vi "Wait for Client.vi"(8 "Error In":errorcluster, 9 "userInfo":T1, 10 "workspace":T2={"x"=200.0, "y"=200.0, "z"=0.0}, 11 "Local TCP Port":u16=32123) -> (0 "Error Out":errorcluster, 3 "Connection":T3={"UDP Connection ID"=refnum, "TCP Connection ID"=refnum, "Remote UDP Port"=61557, "Remote IP"=0})   [LabVIEW 2017, in "Game.lvlib" / "GameComms.lvlib"]
uses:
  GameComms.lvlib
  TypeDefs/Connection.ctl
  TypeDefs/WorkspaceConfig.ctl
  TypeDefs/UserInfo.ctl
  TypeDefs/TCP UDP Ref FGV Commands.ctl
  TypeDefs/ClientConfigData.ctl
  TypeDefs/ClientNetworkParameters.ctl
  TypeDefs/ServerConfigData.ctl
  TypeDefs/ServerNetworkParameters.ctl
panel:
  out "net address":u32
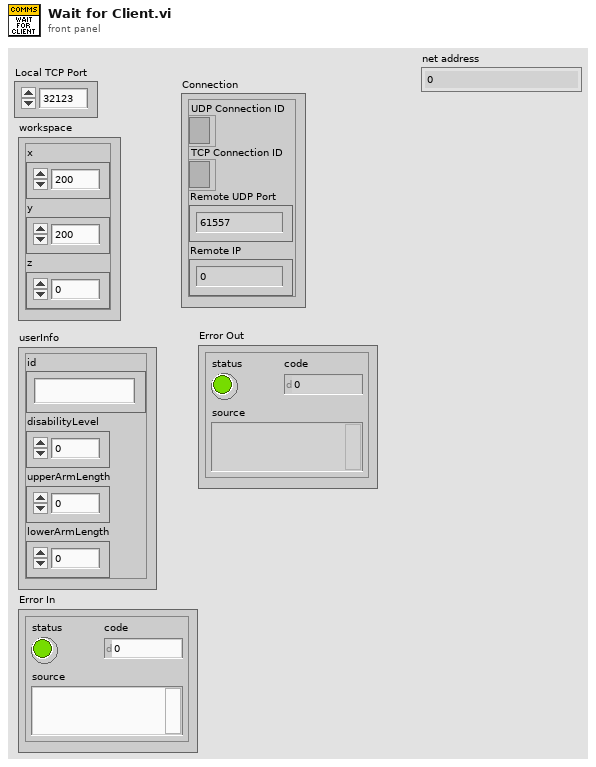
[diagram p1: front panel]
types:
  T1 = typedef "Game.lvlib/GameComms.lvlib/UserInfo.ctl" = cluster{"id":string, "disabilityLevel ":dbl, "upperArmLength":dbl, "lowerArmLength":dbl}
  T2 = typedef "Game.lvlib/GameComms.lvlib/WorkspaceConfig.ctl" = cluster{"x":dbl, "y":dbl, "z":dbl}
  T3 = typedef "Game.lvlib/GameComms.lvlib/Connection.ctl" = cluster{"UDP Connection ID":refnum<k16>, "TCP Connection ID":refnum<k5>, "Remote UDP Port":u16, "Remote IP":u32}
  T4 = enum16{"Standard", "Buffered", "CRLF", "Immediate"}
  T5 = typedef "Game.lvlib/GameComms.lvlib/ServerConfigData.ctl" = cluster{"network":T6, "workspace":T2, "userInfo":T1}
  T6 = typedef "Game.lvlib/GameComms.lvlib/ServerNetworkParameters.ctl" = cluster{"serverUdpPort":u16}
  T7 = typedef "Game.lvlib/GameComms.lvlib/ClientConfigData.ctl" = cluster{"network":T8}
  T8 = typedef "Game.lvlib/GameComms.lvlib/ClientNetworkParameters.ctl" = cluster{"clientUdpPort":u16}
  T9 = typedef "Game.lvlib/GameComms.lvlib/TCP UDP Ref FGV Commands.ctl" = enum16{"Set", "Get"}
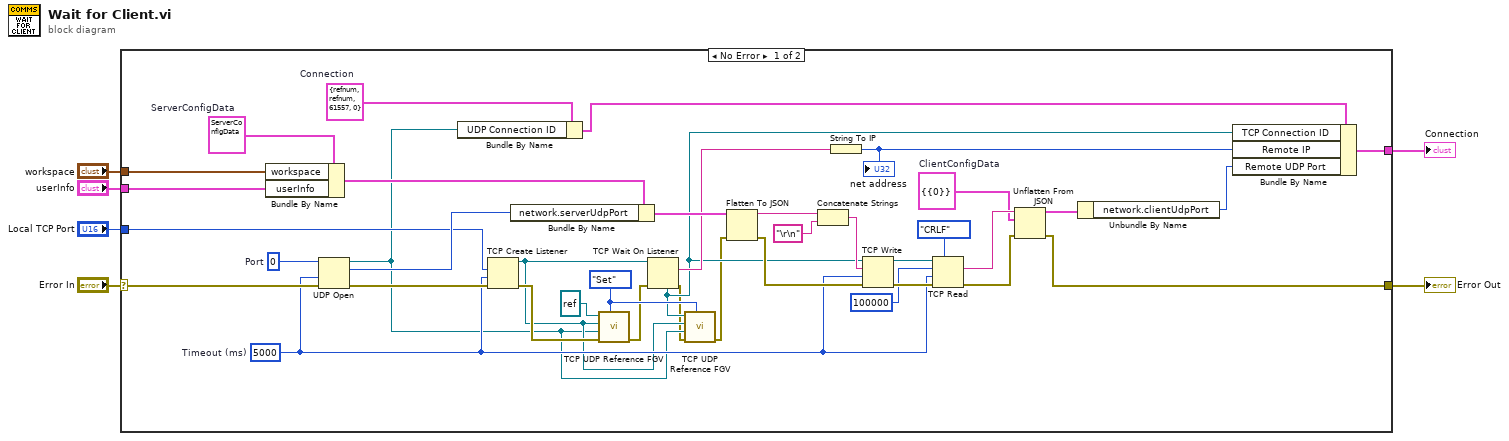
[diagram p0: block diagram]
diagram:
  n1 = case shown="No Error" "Error In" {
    selector: "Error In" -> [w35 w46]
    tunnel: "Local TCP Port" -> [w31 _]
    tunnel: [w24 w46] -> w4
    tunnel: [w18 _] -> w3
    tunnel: "workspace" -> [w16 _]
    tunnel: "userInfo" -> [w14 _]
    frame No Error {
      w17 = T5 {"network"={"serverUdpPort"=0}, "workspace"={"x"=200.0, "y"=200.0, "z"=0.0}, "userInfo"={"id"="", "disabilityLevel "=0.0, "upperArmLength"=0.0, "lowerArmLength"=0.0}}  # ServerConfigData
      w25 = T7 {"network"={"clientUdpPort"=0}}  # ClientConfigData
      w22 = T3 {"UDP Connection ID"=refnum, "TCP Connection ID"=refnum, "Remote UDP Port"=61557, "Remote IP"=0}  # Connection
      w13 = TCP_UDP_Ref_FGV_Commands."Set" ("Command")
      w28 = 5000  # Timeout (ms)
      w36 = u16 0  # Port
      n2 = Bundle By Name(cluster=w17, "workspace"=w16, "userInfo"=w14) -> (w15:T5)
      n3 = UDP Open(8:w35, 9:w28, 11:w36) -> (port=w11:refnum<k16>, 0:w34:errorcluster, 2:w37:u16)  [unwired: 2 in]
      n4 = Bundle By Name(cluster=w22, "UDP Connection ID"=w11) -> (w21:T3)
      n5 = TCP Create Listener(8:w34, 9:w28, 10:w31) -> (0:w33:errorcluster, 3:w12:refnum<k5>)  [unwired: 2 in, 1 out]
      n6 = Bundle By Name(cluster=w15, "network.serverUdpPort"=w37) -> (w30:T5)
      n7 = call "TCP UDP Reference FGV.vi"("Command"=w13, "Error In"=w33, "UDP Connection ID"=w11, "TCP Listener ID"=w12, "TCP Connection ID"=refnum<k5> refnum) -> ("Error Out"=w9:errorcluster)  [unwired: 3 in, 3 out]
      n8 = TCP Wait On Listener(8:w9, 11:w12) -> (0:w8:errorcluster, 2:w29:string, 4:w10:refnum<k5>)  [unwired: 2 in, 2 out]
      n9 = call "TCP UDP Reference FGV.vi"("Command"=w13, "Error In"=w8, "UDP Connection ID"=w11, "TCP Listener ID"=w12, "TCP Connection ID"=w10) -> ("Error Out"=w7:errorcluster)  [unwired: 3 in, 3 out]
      n10 = Flatten To JSON(anything=w30, error in (no error)=w7) -> (JSON string=w40:string, 11:w45:errorcluster)  [unwired: 1 in]
      n11 = Concatenate Strings(w40, "\r\n" ("string")) -> (w39:string)
      n12 = String To IP(1:w29) -> (0:w20:u32)
      "net address" <- w20
      n13 = TCP Write(connection ID=w10, data in=w39, error in (no error)=w45, 9:w28) -> (connection ID out=w43:refnum<k5>, error out=w44:errorcluster)  [unwired: 1 out]
      n14 = TCP Read(connection ID=w43, bytes to read=100000, error in (no error)=w44, 7:T4."CRLF" ("mode (standard)"), 9:w28) -> (data out=w26:string, error out=w27:errorcluster)  [unwired: 1 out]
      n15 = Unflatten From JSON(JSON string=w26, type and defaults=w25, error in (no error)=w27) -> (value=w23:T7, error out=w24:errorcluster)  [unwired: 4 in]
      n16 = Unbundle By Name(w23) -> ("network.clientUdpPort"=w19:u16)
      n17 = Bundle By Name(cluster=w21, "TCP Connection ID"=w10, "Remote IP"=w20, "Remote UDP Port"=w19) -> (w18:T3)
    }
    frame Error {
    }
  }
  "Error Out" <- w4
  "Connection" <- w3
